vi "checkArrSizeWithIdxArr.vi"(8 "error in (no error)":errorcluster, 10 "Idx Array":i32[](array[numeric]), 11 "Array Size":i32) -> (0 "error out":errorcluster, 3 "In Spec":bool)   [LabVIEW 2016]
doc: "Check the element in index array is in the spec of array size or not."
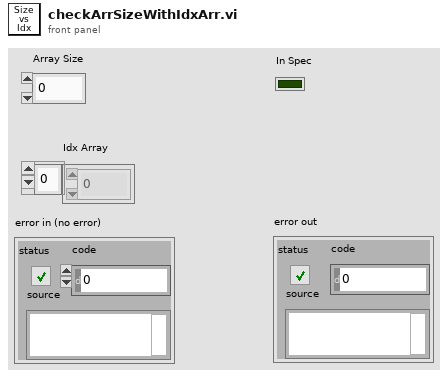
[diagram p1: front panel]
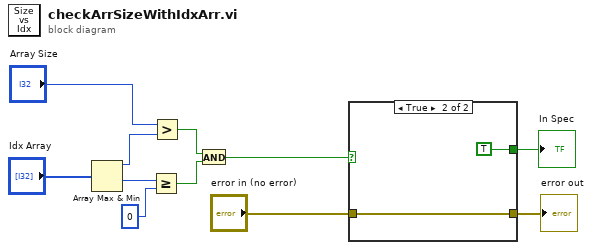
[diagram p0: block diagram]
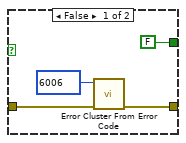
[diagram p2: hidden frame]
diagram:
  n1 = Array Max & Min(array="Idx Array") -> (max value=w10:i32, min value=w9:i32)  [unwired: 2 out]
  n2 = Greater Or Equal?(x=w9, y=0) -> (x >= y?=w6:bool)
  n3 = Greater?(x="Array Size", y=w10) -> (0:w7:bool)
  n4 = And(x=w7, y=w6) -> (x .and. y?=w5:bool)
  n5 = case shown="True" w5 {
    tunnel: [FALSE ("In Spec") TRUE ("In Spec")] -> w4
    tunnel: "error in (no error)" -> [w12 w16]
    tunnel: [w13 w16] -> w2
    frame False {
      n6 = call <vilib>:"Error Cluster From Error Code.vi"("error in (no error)"=w12, "error code (0)"=6006 ("code")) -> ("error out"=w13:errorcluster)  [unwired: 7 in]
    }
    frame True {
    }
  }
  "In Spec" <- w4
  "error out" <- w2
